vi "Draw Named Glyph.vi"(4 "Size":dbl=16.0, 5 "Transform (Center)":refnum<class "Transform.lvclass">, 6 "Colors":T1={"Front"={"Color"=0, "Alpha"=255}, "Back"={"Color"=16448250, "Alpha"=255}}, 7 "Glyph Source in":refnum<class "Glyph Source.lvclass">, 8 "error in (no error)":errorcluster, 9 "Glyph Name":string, 10 "Glyph Drawer in":refnum<class "Glyph Drawer.lvclass">, 11 "Glyph Canvas in":refnum<class "Glyph Canvas.lvclass">) -> (0 "error out":errorcluster, 2 "Glyph Drawer out":refnum<class "Glyph Drawer.lvclass">, 3 "Glyph Canvas out":refnum<class "Glyph Canvas.lvclass">)   [LabVIEW 2023, in "Font Glyph Drawer Interface.lvlib" / "Glyph Canvas.lvclass"]
uses:
  Glyph Canvas.lvclass
  Glyph Drawer/Glyph Drawer.lvclass
  Glyph Source/Glyph Source.lvclass
  Transform/Transform.lvclass
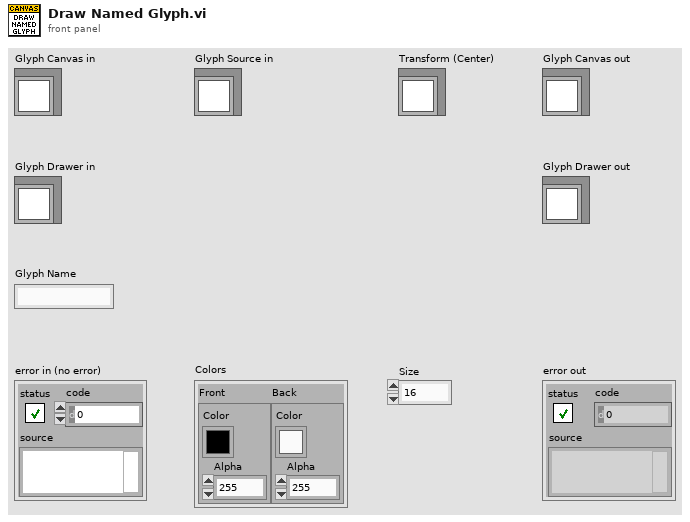
[diagram p1: front panel]
types:
  T1 = cluster{"Front":cluster{"Color":u32, "Alpha":u8}, "Back":cluster{"Color":u32, "Alpha":u8}}
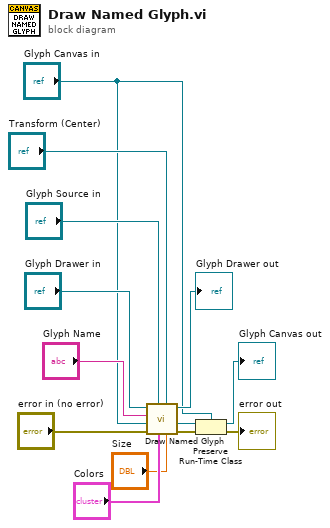
[diagram p0: block diagram]
diagram:
  n1 = call "Draw Named Glyph.vi"("Size"="Size", "Transform (Center)"="Transform (Center)", "Colors"="Colors", "Glyph Source in"="Glyph Source in", "error in (no error)"="error in (no error)", "Destination"="Glyph Canvas in", "Glyph Name"="Glyph Name", "Glyph Drawer in"="Glyph Drawer in") -> ("error out"=w12:errorcluster, "Destination Out"=w4:refnum<class "Glyph Canvas.lvclass">, "Glyph Drawer out"=→"Glyph Drawer out":refnum<class "Glyph Drawer.lvclass">)  [unwired: 1 in]
  n2 = Preserve Run-Time Class(object in=w4, error in=w12, 2:"Glyph Canvas in") -> (object out=→"Glyph Canvas out":refnum<class "Glyph Canvas.lvclass">, error out=→"error out":errorcluster)
